vi "CreateGyroOutput.vi"(10 "MessageCounter":u8, 11 "MockGyroData":T1={"BufferUpdateFIFO"="MockGyroBufferUpdate", "MockGyroCommandInput"="ModbusSubnetEGyroRxDataFIFO", "MockGyroDataOutput"="ModbusSubnetEGyroTxDataFIFO", "MockGyroDataRate"="MockGyroDataRateRegister", "MockGyroXValue"="MockGyroXValueRegister", "MockGyroYValue"="MockGyroYValueRegister", "MockGyroZValue"="MockGyroZValueRegister", "MockGyroStatus"="MockGyroStatusRegister", "MockGyroTemperature"="MockGyroTemperatureRegister", "CRCDataFIFO"="MockGyroCRCDataFIFO", "CRCCalculateFIFO"="MockGyroCRCCalculateFIFO", "CRCFIFO"="MockGyroCRCFIFO", "MockGyroCommandReplyFIFO"="MockGyroCommandReplyFIFO", "MockGyroReplyReadyFIFO"="MockGyroReplyReadyFIFO", "MockGyroModeFIFO"="MockGyroModeFIFO"}) -> (3 "DataMessage":u8[](array[numeric]))   [LabVIEW 2016]
uses:
  <vilib>/rvi/DataTransferAndStorage/Container/XNode/niFpgaContainer.xnode
  FPGAMockGyro.lvlib
  <vilib>/rvi/Memory/Memory_Emulation/nirvimemoryFastEmulation.vi
  <vilib>/rvi/Memory/Memory_Emulation/nirvimemoryEmulation.vi
  DataTypes/MockGyroData.ctl
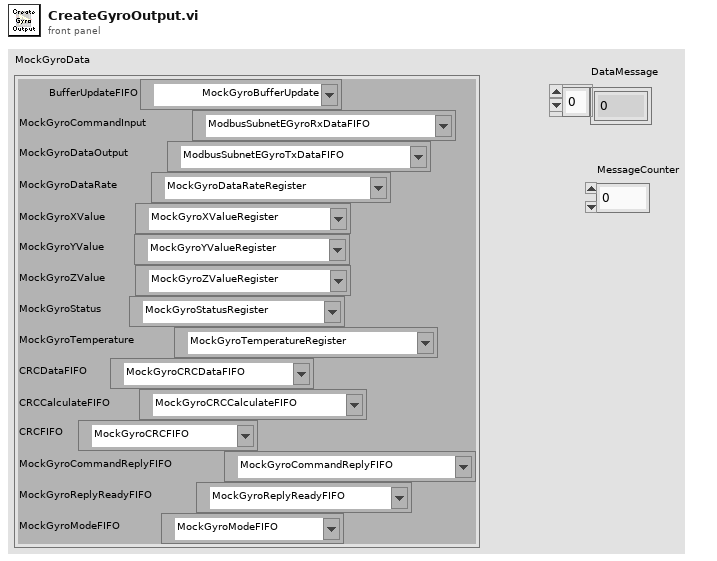
[diagram p1: front panel]
types:
  T1 = typedef "FPGAMockGyro.lvlib/MockGyroData.ctl" = cluster{"BufferUpdateFIFO":refnum<k21>, "MockGyroCommandInput":refnum<k21>, "MockGyroDataOutput":refnum<k21>, "MockGyroDataRate":refnum<k21>, "MockGyroXValue":refnum<k21>, "MockGyroYValue":refnum<k21>, "MockGyroZValue":refnum<k21>, "MockGyroStatus":refnum<k21>, "MockGyroTemperature":refnum<k21>, "CRCDataFIFO":refnum<k21>, "CRCCalculateFIFO":refnum<k21>, "CRCFIFO":refnum<k21>, "MockGyroCommandReplyFIFO":refnum<k21>, "MockGyroReplyReadyFIFO":refnum<k21>, "MockGyroModeFIFO":refnum<k21>}
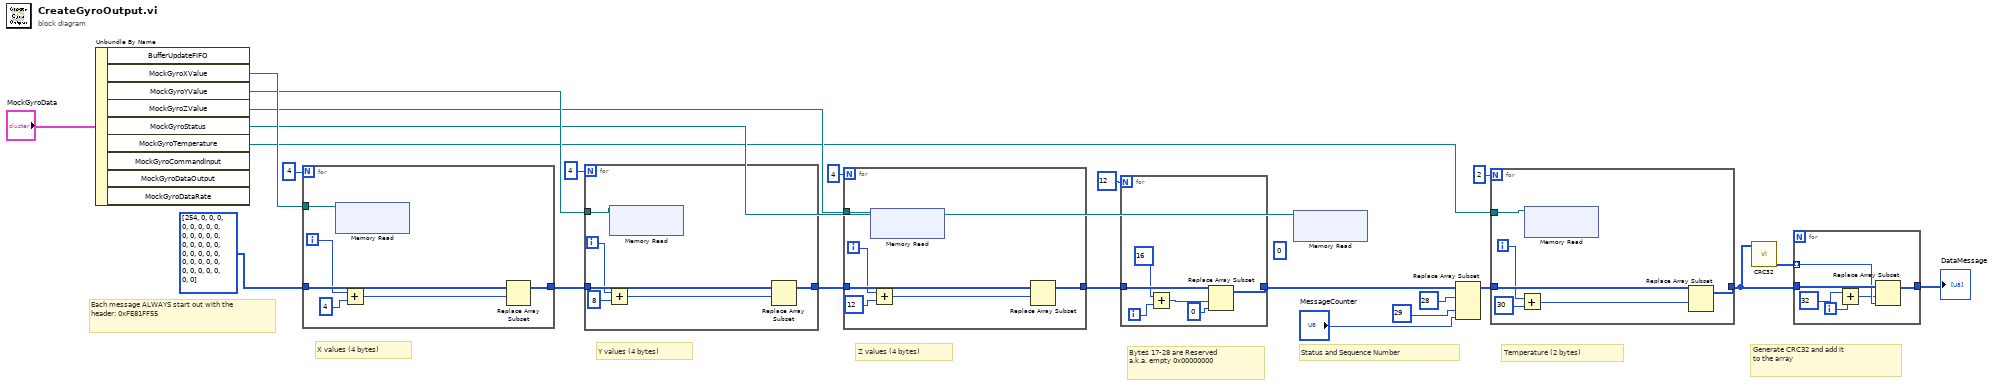
[diagram p0: block diagram]
diagram:
  w12 = u32 0 ("Address")
  # "Generate CRC32 and add it \nto the array"
  # "Temperature (2 bytes)"
  # "Z values (4 bytes)"
  # "Y values (4 bytes)"
  # "X values (4 bytes)"
  # "Status and Sequence Number"
  # "Bytes 17-28 are Reserved\na.k.a. empty 0x00000000"
  # "Each message ALWAYS start out with the header: 0xFE81FF55"
  n1 = Unbundle By Name("MockGyroData") -> ("MockGyroXValue"=w24:refnum<k21>, "MockGyroYValue"=w21:refnum<k21>, "MockGyroZValue"=w17:refnum<k21>, "MockGyroStatus"=w13:refnum<k21>, "MockGyroTemperature"=w8:refnum<k21>)  [unwired: 4 out]
  n2 = for {
    N: 4 -> [_]
    tunnel: w24 -> [w32]
    tunnel: u8[] [254, 0, 0, 0, 0, 0, 0, 0, 0, 0, 0, 0, 0, 0, 0, 0, 0, 0, 0, 0, 0, 0, 0, 0, 0, 0, 0, 0, 0, 0, 0, 0, 0, 0, 0, 0] -> [w29]
    tunnel: [w31] -> w19
    i -> [w28]
    n3 = xnode ("Memory Read")("Memory In"=w32) -> ()  [unwired: 1 out]
    n4 = Add(x=w28, y=4) -> (x+y=w26:i32)
    n5 = Replace Array Subset(array=w29, index=w26) -> (w31:u8[], new element=w30:u8)
  }
  n6 = for {
    N: 4 -> [_]
    tunnel: w21 -> [w39]
    tunnel: w19 -> [w38]
    tunnel: [w37] -> w16
    i -> [w35]
    n7 = Add(x=w35, y=8) -> (x+y=w33:i32)
    n8 = xnode ("Memory Read")("Memory In"=w39) -> ()  [unwired: 1 out]
    n9 = Replace Array Subset(array=w38, index=w33) -> (w37:u8[], new element=w36:u8)
  }
  n10 = for {
    N: 4 -> [_]
    tunnel: w17 -> [w46]
    tunnel: w16 -> [w45]
    tunnel: [w43] -> w14
    i -> [w42]
    n11 = xnode ("Memory Read")("Memory In"=w46) -> ()  [unwired: 1 out]
    n12 = Add(x=w42, y=12) -> (x+y=w40:i32)
    n13 = Replace Array Subset(array=w45, index=w40) -> (w43:u8[], new element=w44:u8)
  }
  n14 = for {
    N: 12 -> [_]
    tunnel: w14 -> [w51]
    tunnel: [w50] -> w11
    i -> [w49]
    n15 = Add(x=16, y=w49) -> (x+y=w47:i32)
    n16 = Replace Array Subset(array=w51, new element=u8 0 ("new element/subarray"), index=w47) -> (w50:u8[])
  }
  n17 = xnode ("Memory Read")("Memory In"=w13) -> ()  [unwired: 1 out]
  n18 = Replace Array Subset(array=w11, index #1=28 ("index"), new element #2="MessageCounter", index #2=29 ("index")) -> (w9:u8[], new element #1=w10:u8)
  n19 = for {
    N: 2 -> [_]
    tunnel: w8 -> [w59]
    tunnel: w9 -> [w58]
    tunnel: [w57] -> w5
    i -> [w55]
    n20 = Add(x=w55, y=30) -> (x+y=w53:i32)
    n21 = xnode ("Memory Read")("Memory In"=w59) -> ()  [unwired: 1 out]
    n22 = Replace Array Subset(array=w58, index=w53) -> (w57:u8[], new element=w56:u8)
  }
  n23 = call "CRC32.vi"("ByteArrayIn"=w5) -> ("CRCByteArray"=w6:u8[])  [unwired: 9 in, 1 out]
  n24 = for {
    tunnel: w6 -> [w63] mode=indexing
    tunnel: w5 -> [w65]
    tunnel: [w64] -> w4
    i -> [w62]
    n25 = Add(x=32, y=w62) -> (x+y=w60:i32)
    n26 = Replace Array Subset(array=w65, new element=w63, index=w60) -> (w64:u8[])
  }
  "DataMessage" <- w4
